vi "ProcessData.vi"(8 "error in (no error)":errorcluster, 9 "State":T1, 10 "Analog Data":T3, 11 "TrialBasedExperiment in":refnum<class "TrialBasedExperiment.lvclass">) -> (0 "error out":errorcluster, 1 "Fixated":bool, 2 "Trigger":T2=enum."Broke Fixation", 3 "TrialBasedExperiment out":refnum<class "TrialBasedExperiment.lvclass">)   [LabVIEW 2014, in "AcquisitionCoreObjects.lvlib" / "TrialBasedExperiment.lvclass"]
uses:
  TrialBasedExperiment.lvclass
  Core SubVIs/Controls/TYPE - Analog Data.ctl
  Trial Based Experiment.lvsc/Trigger.ctl
  Trial Based Experiment.lvsc/State.ctl
  <vilib>/measure/madcrms.llb/Basic Averaged DC-RMS for 1 Chan.vi
  Trial Based Experiment.lvsc
  Core SubVIs/Core SubVIs.lvlib
  <vilib>/measure/NI_MAPro.lvlib
  Acquisition/BehaviorData/BehaviorData.lvclass
panel:
  in  "Incorrect":bool
  in  "Correct":bool
  in  "Toggle Fixation":bool
  in  "Radius":dbl
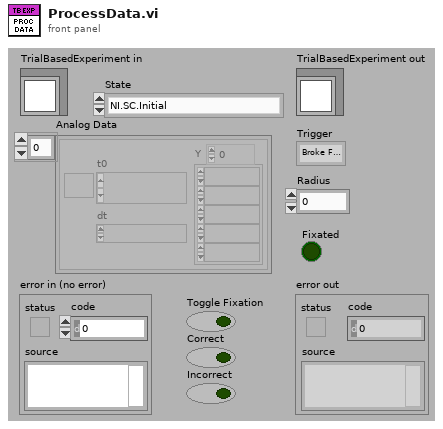
[diagram p1: front panel]
types:
  T1 = typedef "Trial Based Experiment.lvsc/State.ctl" = enum16{"NI.SC.Initial", "NI.SC.History", "NI.SC.ShallowHistory", "NI.SC.Terminal", "Cleanup", "State", "State\\Region\\Pause", "State\\Region\\Response Period", "State\\Region\\Delay Period", "State\\Region\\Hold Fixation", "State\\Region\\Acquire Fixation", "State\\Region\\Abort Trial", "State\\Region\\End Trial", "State\\Region\\Intertrial", "State\\Region\\Start Trial"}
  T2 = typedef "Trial Based Experiment.lvsc/Trigger.ctl" = enum16{"NULL", "Fixated", "Broke Fixation", "Stop", "Correct Response", "Incorrect Response", "Timeout"}
  T3 = typedef "Core SubVIs.lvlib/TYPE - Analog Data.ctl" = waveform(dbl)[]
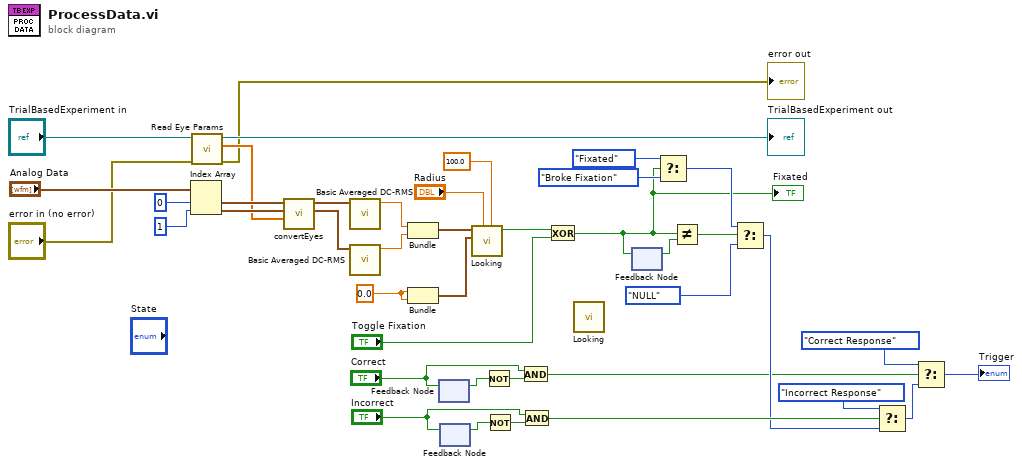
[diagram p0: block diagram]
diagram:
  w4 = 0.0
  n1 = Index Array(array="Analog Data", index #1=0 ("index"), index #2=1 ("index")) -> (element #1=w39:waveform(dbl), element #2=w38:waveform(dbl))
  n2 = call-dynamic "Read Eye Params.vi"("error in (no error)"="error in (no error)", "TrialBasedExperiment in"="TrialBasedExperiment in") -> ("error out"=→"error out":errorcluster, "Eye Params"=w26:dbl[], "TrialBasedExperiment out"=→"TrialBasedExperiment out":refnum<class "TrialBasedExperiment.lvclass">)  [unwired: 7 in]
  n3 = call "convertEyes.vi"("Params"=w26, "Vertical"=w38, "Horizontal"=w39) -> ("Vertical Calibrated"=w36:waveform(dbl), "Horizontal Calibrated"=w37:waveform(dbl))  [unwired: 7 in]
  n4 = call-poly <vilib>:"Basic Averaged DC-RMS.vi"("signal in"=w37) -> ("DC value"=w10:dbl)  [unwired: 7 in, 3 out]
  n5 = call-poly <vilib>:"Basic Averaged DC-RMS.vi"("signal in"=w36) -> ("DC value"=w9:dbl)  [unwired: 7 in, 3 out]
  n6 = Bundle("DC value"=w10, "DC value"=w9) -> (w8:cluster{"DC value":dbl, "DC value":dbl})  [unwired: 1 in]
  n7 = Bundle(w4, w4) -> (w5:cluster{dbl, dbl})  [unwired: 1 in]
  n8 = feedback #1() -> (w23:bool)  [unwired: 1 in]
  n9 = feedback-in #1("Correct") -> ()
  n10 = feedback #2() -> (w20:bool)  [unwired: 1 in]
  n11 = feedback-in #2("Incorrect") -> ()
  n12 = call "Looking.vi"("Break Timeout (ms)"=100.0, "Fixation Radius (px)"="Radius", "Desired Position"=w5, "Eye Position"=w8) -> ("Looking"=w2:bool)  [unwired: 6 in, 1 out]
  n13 = Not(x=w23) -> (.not. x?=w22:bool)
  n14 = Not(x=w20) -> (.not. x?=w19:bool)
  n15 = And(x="Correct", y=w22) -> (x .and. y?=w15:bool)
  n16 = And(x="Incorrect", y=w19) -> (x .and. y?=w17:bool)
  n17 = Exclusive Or(1:"Toggle Fixation", 2:w2) -> (0:w1:bool)
  "Fixated" <- w1
  n18 = call "Looking.vi"() -> ()  [unwired: 10 in, 2 out]
  n19 = feedback #3() -> (w35:bool)  [unwired: 1 in]
  n20 = feedback-in #3(w1) -> ()
  n21 = Select(t=Trigger."Fixated" ("Trigger"), s=w1, f=Trigger."Broke Fixation" ("Trigger")) -> (s? t:f=w32:T2)
  n22 = Not Equal?(x=w1, y=w35) -> (x != y?=w34:bool)
  n23 = Select(t=w32, s=w34, f=Trigger."NULL" ("Trigger")) -> (s? t:f=w16:T2)
  n24 = Select(t=Trigger."Incorrect Response", s=w17, f=w16) -> (s? t:f=w14:T2)
  n25 = Select(t=Trigger."Correct Response", s=w15, f=w14) -> (s? t:f=→"Trigger":T2)
